vi "CRYPIC Save StepView.vi"(7 "sAction":string, 10 "tFrame":T2) -> (2 "tFrame_Out":T2)   [LabVIEW 2013]
uses:
  <vilib>/Utility/miscctls.llb/LVRectTypeDef.ctl
  CRYMain Sub Window Global.vi
panel:
  in  "bWait":bool=TRUE
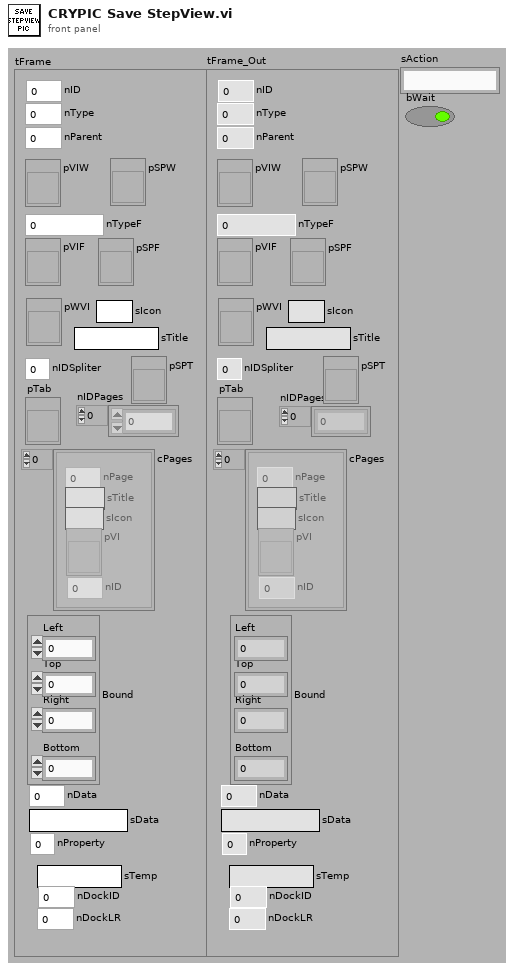
[diagram p1: front panel]
types:
  T1 = typedef "LVRectTypeDef.ctl" = cluster{"Left":i16, "Top":i16, "Right":i16, "Bottom":i16}
  T2 = cluster{"nType":i32, "nParent":i32, "pVIW":refnum<vi>, "pSPW":refnum<vi>, "nTypeF":i32, "pVIF":refnum<vi>, "pSPF":refnum<vi>, "nIDSpliter":i32, "nProperty":i32, "Bound":T1, "nID":i32, "nData":i32, "sData":string, "pWVI":refnum<vi>, "sTitle":string, "cPages":cluster{"nPage":i32, "sTitle":string, "sIcon":string, "pVI":refnum<vi>, "nID":i32}[], "pTab":refnum<vi>, "nIDPages":i32[], "pSPT":refnum<vi>, "sTemp":string, "nDockID":i32, "nDockLR":i32, "sIcon":string}
  T3 = cluster{"CLOSE_HIDE":i32, "CLOSE_CLOSE":i32, "DOCK_ENABLE":i32, "DOCK_DISABLE":i32, "FOCUS_SHOW":i32, "FOCUS_HIDE":i32}
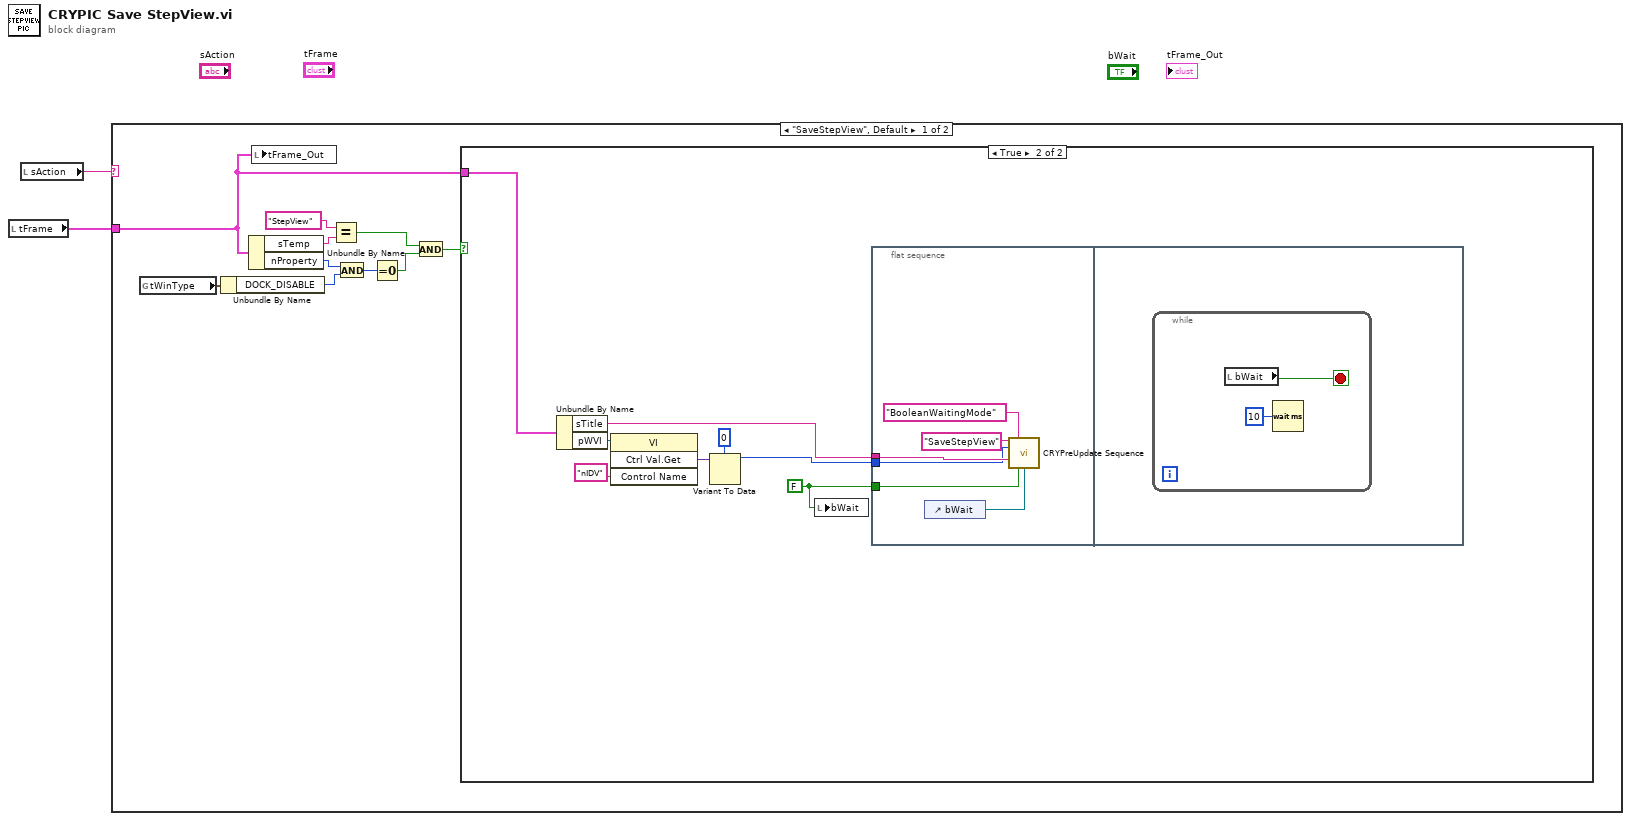
[diagram p0: block diagram]
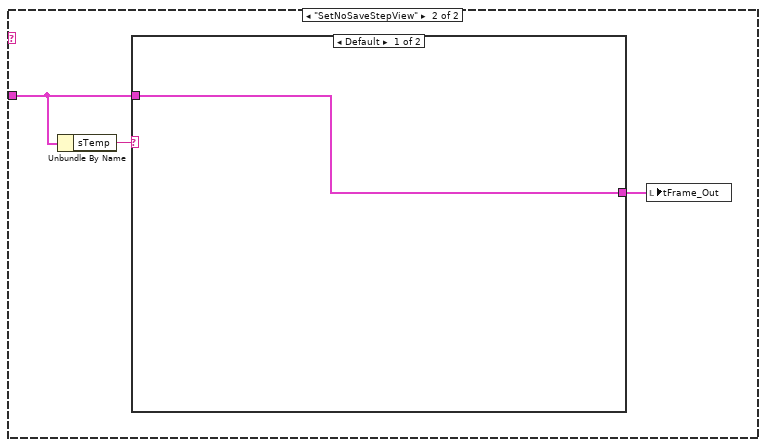
[diagram p3: hidden frame]
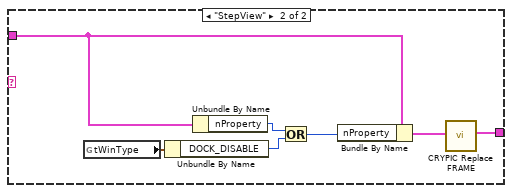
[diagram p4: hidden frame]
diagram:
  n1 = local read "tFrame"() -> (w2:T2)
  n2 = local read "sAction"() -> (w1:string)
  n3 = case shown="\"SaveStepView\", Default" w1 {
    tunnel: w2 -> [w3 w30]
    frame "SaveStepView", Default {
      n4 = global read "CRYMain Sub Window Global.vi" "tWinType"() -> (w12:T3)
      n5 = Unbundle By Name(w12) -> ("DOCK_DISABLE"=w10:i32)
      n6 = Unbundle By Name(w3) -> ("sTemp"=w8:string, "nProperty"=w11:i32)
      n7 = local write "tFrame_Out"(w3) -> ()
      n8 = Equal?(x="StepView", y=w8) -> (x = y?=w6:bool)
      n9 = And(x=w11, y=w10) -> (x .and. y?=w7:i32)
      n10 = Equal To 0?(x=w7) -> (x = 0?=w5:bool)
      n11 = And(x=w6, y=w5) -> (x .and. y?=w4:bool)
      n12 = case shown="True" w4 {
        tunnel: w3 -> [_ w18]
        frame False {
        }
        frame True {
          w13 = FALSE
          n13 = Unbundle By Name(w18) -> ("sTitle"=w15:string, "pWVI"=w17:refnum<vi>)
          n14 = invoke class="VI" method="Ctrl Val.Get"(reference=w17, "Control Name"="nIDV") -> ("Get Control Value Variant"=w20:variant)  [unwired: 2 in, 3 out]
          n15 = Variant To Data(type=0, Variant=w20) -> (data=w14:i32)  [unwired: 1 in, 1 out]
          n16 = local write "bWait"(w13) -> ()
          n17 = flat-sequence {
            tunnel: w15 -> [w24]
            tunnel: w14 -> [w23]
            tunnel: w13 -> [w22]
            frame #0 {
              n18 = control-ref of="bWait"() -> (w21:refnum<vi>)
              n19 = call "CRYPreUpdate Sequence.vi"("EventName"="SaveStepView", "Mode"="BooleanWaitingMode", "Proper VI No"=w23, "Project View Step Name Identifier Arg1"=w24, "AllChangeFlg"=w22, "Ref Variant"=w21) -> ()  [unwired: 10 in]
            }
            frame #1 {
              n20 = while {
                stop <- w27 stop-if-true
                n21 = local read "bWait"() -> (w27:bool)
                n22 = Wait (ms)(milliseconds to wait=u32 10) -> ()  [unwired: 1 out]
              }
            }
          }
        }
      }
    }
    frame "SetNoSaveStepView" {
      n23 = Unbundle By Name(w30) -> ("sTemp"=w29:string)
      n24 = case shown="Default" w29 {
        tunnel: w30 -> [w32 w36]
        tunnel: [w32 w33] -> w31
        frame Default {
        }
        frame "StepView" {
          n25 = global read "CRYMain Sub Window Global.vi" "tWinType"() -> (w39:T3)
          n26 = Unbundle By Name(w39) -> ("DOCK_DISABLE"=w37:i32)
          n27 = Unbundle By Name(w36) -> ("nProperty"=w38:i32)
          n28 = Or(x=w38, y=w37) -> (x .or. y?=w35:i32)
          n29 = Bundle By Name(cluster=w36, "nProperty"=w35) -> (w34:T2)
          n30 = call "CRYPIC Replace FRAME.vi"("tFrame"=w34) -> ("tFrame_Out"=w33:T2)  [unwired: 10 in]
        }
      }
      n31 = local write "tFrame_Out"(w31) -> ()
    }
  }
